vi "POP_Close.vi"(7 "Name":string, 8 "error in (no error)":errorcluster) -> (0 "error out":errorcluster)   [LabVIEW 2016]
uses:
  Private/Ctrls/POP_Popup Operation.ctl
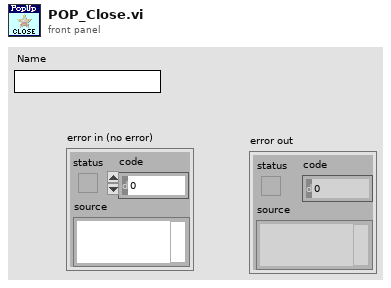
[diagram p1: front panel]
types:
  T1 = typedef "POP_Popup Operation.ctl" = enum16{"Show", "Initialize", "Close", "Popup Done", "Register a Location's Type", "Retrieve Location's Type"}
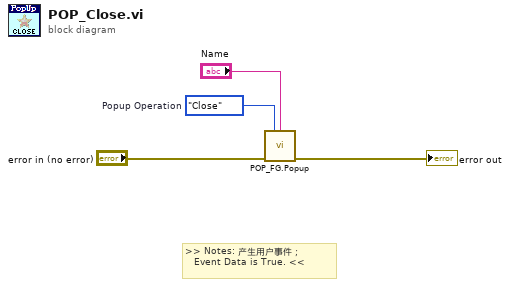
[diagram p0: block diagram]
diagram:
  w4 = POP_Popup_Operation."Close"  # Popup Operation
  # ">> Notes: 产生用户事件；\n   Event Data is True. <<"
  n1 = call "POP_FG.Popup.vi"("Popup Operation"=w4, "Name"="Name", "Error In"="error in (no error)") -> ("Error Out"=→"error out":errorcluster)  [unwired: 9 in, 3 out]
